vi "DeInit Done.vi"(8 "error in (no error)":errorcluster, 10 "InstrumentData":T1, 11 "SpectroscopyUI in":refnum<class "SpectroscopyUI.lvclass">) -> (0 "error out":errorcluster, 3 "SpectroscopyUI out":refnum<class "SpectroscopyUI.lvclass">)   [LabVIEW 2023, in "SpectroscopyUI.lvlib" / "SpectroscopyUI.lvclass"]
uses:
  SpectroscopyUI.lvclass
  SpectroscopyUI.lvclass/SpectroscopyUI.ctl
  typedefs/instrumentType.ctl
  typedefs/typedefs.lvlib
  <vilib>/ActorFramework/Message Enqueuer/Message Enqueuer.lvclass
  typedefs/InstrumentData.ctl
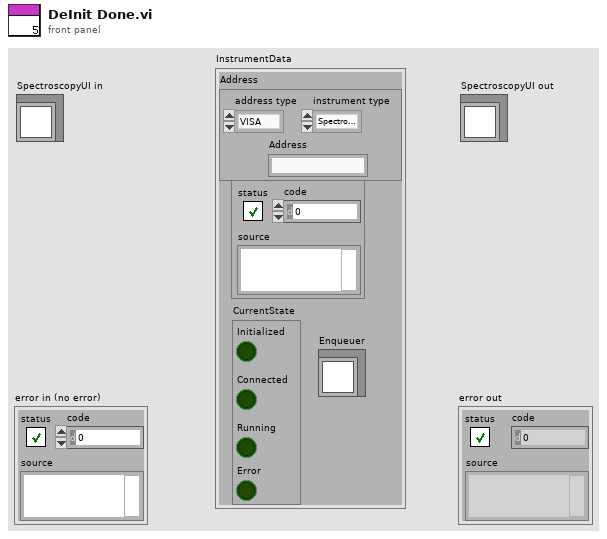
[diagram p1: front panel]
types:
  T1 = typedef "typedefs.lvlib/InstrumentData.ctl" = cluster{"Instr Error":errorcluster, "Address":cluster{"address type":enum16{"VISA", "Index"}, "Address":string, "instrument type":T2}, "CurrentState":cluster{"Initialized":bool, "Connected":bool, "Running":bool, "Error":bool}, "Enqueuer":refnum<class "Message Enqueuer.lvclass">}
  T2 = typedef "typedefs.lvlib/instrumentType.ctl" = enum16{"Spectrometer", "Camera", "Stepper"}
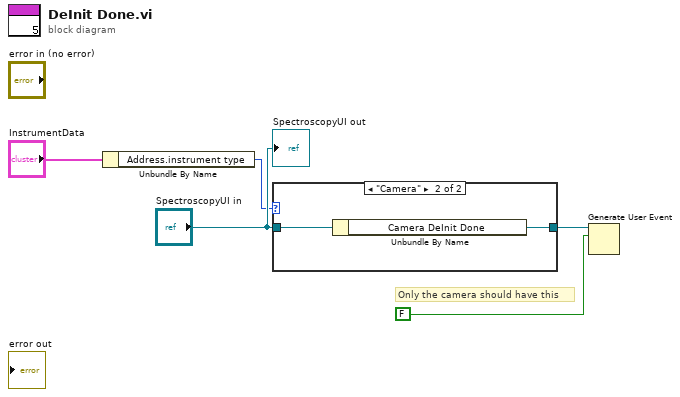
[diagram p0: block diagram]
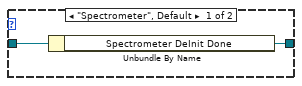
[diagram p2: hidden frame]
diagram:
  # "Only the camera should have this"
  n1 = Unbundle By Name("InstrumentData") -> ("Address.instrument type"=w1:T2)
  n2 = case shown="\"Camera\"" w1 {
    tunnel: "SpectroscopyUI in" -> [w6 w9]
    tunnel: [w7 w8] -> w4
    frame "Spectrometer", Default {
      n3 = Unbundle By Name(w6) -> ("Spectrometer DeInit Done"=w7:refnum<user-event>)
    }
    frame "Camera" {
      n4 = Unbundle By Name(w9) -> ("Camera DeInit Done"=w8:refnum<user-event>)
    }
  }
  n5 = Generate User Event(user event=w4, event data cluster=FALSE ("event data")) -> ()  [unwired: 2 in, 2 out]
  "SpectroscopyUI out" <- "SpectroscopyUI in"
